vi "Add AWGN.vi"(8 "Add AWGN?":bool=TRUE, 10 "SNR [dB]":dbl, 11 "Input":cluster{"t0":dbl, "dt":dbl, "Y":cdb[]}={"t0"=0.0, "dt"=1.0, "Y"=[]} caption="input waveform" {"Y" format="%.3f"; "dt" format="%^.2e"; "t0" format="%.4f"}) -> (3 "Output":cluster{"t0":dbl, "dt":dbl, "Y":cdb[]}={"t0"=0.0, "dt"=1.0, "Y"=[]} caption="output waveform" {"Y" format="%.3f"; "dt" format="%^.2e"; "t0" format="%.4f"})   [LabVIEW 2011]
uses:
  <vilib>/Analysis/NI_AALBase.lvlib
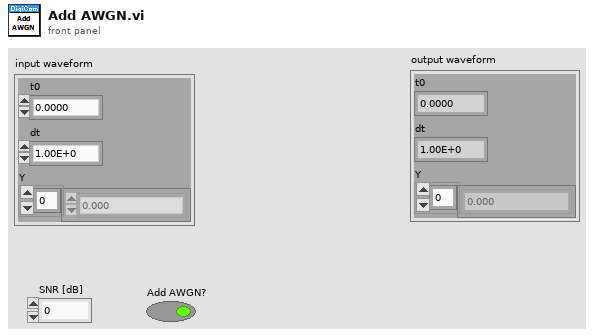
[diagram p1: front panel]
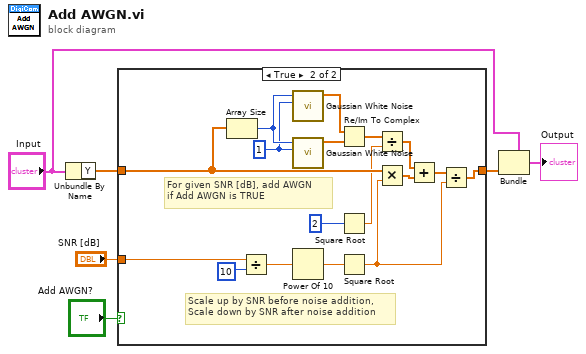
[diagram p0: block diagram]
diagram:
  n1 = Unbundle By Name("Input") -> ("Y"=w2:cdb[])
  n2 = case shown="True" "Add AWGN?" {
    tunnel: "SNR [dB]" -> [_ w24]
    tunnel: w2 -> [w7 w17]
    tunnel: [w7 w13] -> w1
    frame False {
    }
    frame True {
      w12 = 1
      # "Scale up by SNR before noise addition,\nScale down by SNR after noise addition"
      # "For given SNR [dB], add AWGN\nif Add AWGN is TRUE"
      n3 = Array Size(array=w17) -> (size(s)=w20:i32)
      n4 = Divide(x=w24, y=10) -> (x/y=w22:dbl)
      n5 = call <vilib>:"Gaussian White Noise.vi"("standard deviation"=w12, "samples"=w20) -> ("Gaussian noise pattern"=w19:dbl[])  [unwired: 8 in, 1 out]
      n6 = call <vilib>:"Gaussian White Noise.vi"("standard deviation"=w12, "samples"=w20) -> ("Gaussian noise pattern"=w18:dbl[])  [unwired: 8 in, 1 out]
      n7 = Power Of 10(x=w22) -> (10^x=w21:dbl)
      n8 = Re/Im To Complex(1:w18, 2:w19) -> (0:w11:cdb[])
      n9 = Square Root(x=2) -> (sqrt(x)=w10:dbl)
      n10 = Square Root(x=w21) -> (sqrt(x)=w16:dbl)
      n11 = Divide(x=w11, y=w10) -> (x/y=w8:cdb[])
      n12 = Multiply(x=w17, y=w16) -> (x*y=w15:cdb[])
      n13 = Add(x=w8, y=w15) -> (x+y=w14:cdb[])
      n14 = Divide(x=w14, y=w16) -> (x/y=w13:cdb[])
    }
  }
  n15 = Bundle(cluster="Input", "Y"=w1) -> (→"Output":cluster{"t0":dbl, "dt":dbl, "Y":cdb[]})  [unwired: 2 in]
